vi "TESTE.vi"() -> ()   [LabVIEW 2014]
panel:
  in  "Boolean 2":bool
  out "Boolean":bool
  in  "Thermometer":dbl(slide) scale=0.0..100.0
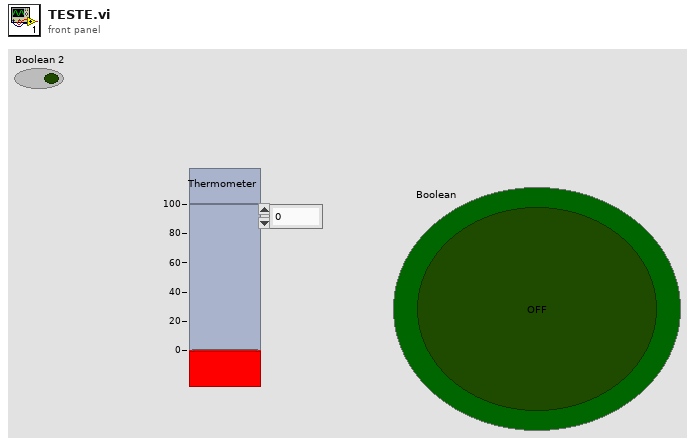
[diagram p1: front panel]
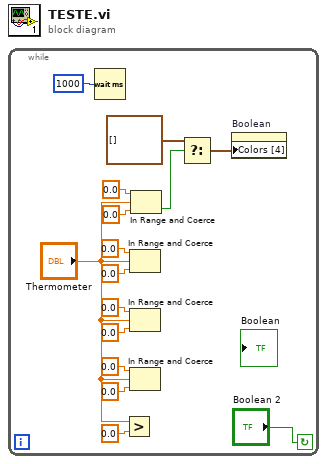
[diagram p0: block diagram]
diagram:
  n1 = while {
    stop <- "Boolean 2" continue-if-true
    n2 = Wait (ms)(milliseconds to wait=u32 1000 ("millisecond timer value")) -> ()  [unwired: 1 out]
    n3 = Greater?(x="Thermometer", y=0.0 ("x")) -> ()  [unwired: 1 out]
    n4 = In Range and Coerce(upper limit=0.0 ("x"), x="Thermometer", lower limit=0.0 ("x")) -> ()  [unwired: 2 out]
    n5 = In Range and Coerce(upper limit=0.0 ("x"), x="Thermometer", lower limit=0.0 ("x")) -> ()  [unwired: 2 out]
    n6 = In Range and Coerce(upper limit=0.0 ("x"), x="Thermometer", lower limit=0.0 ("x")) -> ()  [unwired: 2 out]
    n7 = In Range and Coerce(upper limit=0.0 ("x"), x="Thermometer", lower limit=0.0 ("x")) -> (In Range?=w5:bool)  [unwired: 1 out]
    n8 = Select(t=cluster{u32, u32}[] [] ("Colors [4]"), s=w5) -> (s? t:f=w3:cluster{u32, u32}[])  [unwired: 1 in]
    n9 = property on="Boolean" class="Bool (strict)"("Colors [4]"=w3) -> ()  [unwired: 2 in, 2 out]
  }
